vi "Relative Kernel Indices.vi"(1 "Kernel":bool[][](array[boolean])=[[TRUE, TRUE, TRUE], [TRUE, FALSE, TRUE], [TRUE, TRUE, TRUE]]) -> (0 "Relative Indices":cluster{"[0]":i32, "[1]":i32}[](array[cluster]))   [LabVIEW 2020, in "VIM Tools.lvlib"]
uses:
  VIM Tools.lvlib
  2f2fffae-2d87-4e9d-8675-a6890f93f1c9.vi
  2f2fffae-2d87-4e9d-8675-a6890f93f1c9.vi/734d14e6-0ce6-406a-83b8-e03d21e7172a.vi
  Unravel Index.vi
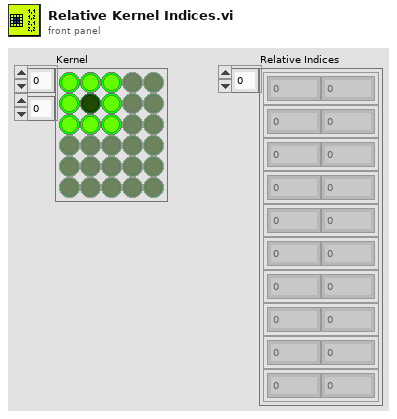
[diagram p1: front panel]
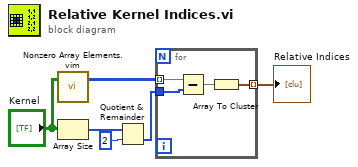
[diagram p0: block diagram]
diagram:
  n1 = call "Nonzero Array Elements.vim"("Array"="Kernel") -> ("ND Index"=w6:i32[][])  [unwired: 1 in, 1 out]
  n2 = Array Size(array="Kernel") -> (size(s)=w4:i32[])
  n3 = Quotient & Remainder(x=w4, y=2) -> (floor(x/y)=w1:i32[])  [unwired: 1 out]
  n4 = for {
    tunnel: w6 -> [w10] mode=indexing
    tunnel: [w7] -> w2 mode=indexing
    tunnel: w1 -> [w8]
    n5 = Subtract(x=w10, y=w8) -> (x-y=w9:i32[])
    n6 = Array To Cluster(array=w9) -> (cluster=w7:cluster{"[0]":i32, "[1]":i32})
  }
  "Relative Indices" <- w2
